vi "PixieCalcCountDataold.vi"(0 "CrsrList":T2, 1 "Histogram Data":u32[][](array[numeric]), 2 "CH0 LT":dbl, 3 "CH1 LT":dbl) -> (5 "Count Data":T1)   [LabVIEW 2011]
uses:
  <vilib>/Utility/miscctls.llb/LVCursorListTypeDef.ctl
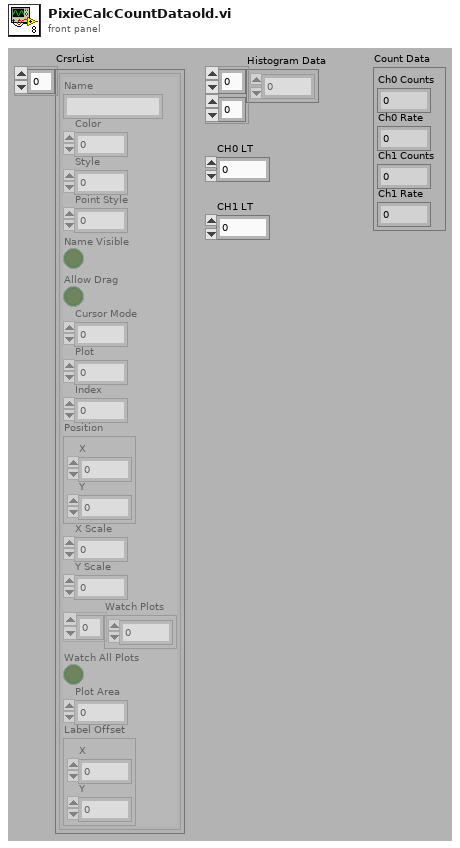
[diagram p1: front panel]
types:
  T1 = cluster{"Ch0 Counts":u32, "Ch0 Rate":dbl, "Ch1 Counts":u32, "Ch1 Rate":dbl}
  T2 = typedef "LVCursorListTypeDef.ctl" = cluster{"Name":string, "Color":u32, "Style":u8, "Point Style":u8, "Name Visible":bool, "Allow Drag":bool, "Cursor Mode":u32, "Plot":i32, "Index":i32, "Position":cluster{"X":dbl, "Y":dbl}, "X Scale":u32, "Y Scale":u32, "Watch Plots":i32[], "Watch All Plots":bool, "Plot Area":i32, "Label Offset":cluster{"X":dbl, "Y":dbl}}[]
  T3 = cluster{"Name":string, "Color":u32, "Style":u8, "Point Style":u8, "Name Visible":bool, "Allow Drag":bool, "Cursor Mode":u32, "Plot":i32, "Index":i32, "Position":cluster{"X":dbl, "Y":dbl}, "X Scale":u32, "Y Scale":u32, "Watch Plots":i32[], "Watch All Plots":bool, "Plot Area":i32, "Label Offset":cluster{"X":dbl, "Y":dbl}}
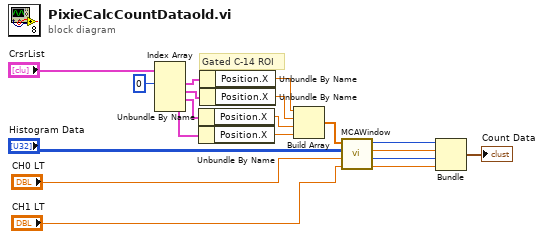
[diagram p0: block diagram]
diagram:
  # "Gated C-14 ROI"
  n1 = Index Array(array="CrsrList", index #1=0 ("index")) -> (element #1=w10:T3, element #2=w11:T3, element #3=w12:T3, element #4=w13:T3)  [unwired: 3 in]
  n2 = Unbundle By Name(w12) -> ("Position.X"=w3:dbl)
  n3 = Unbundle By Name(w13) -> ("Position.X"=w5:dbl)
  n4 = Unbundle By Name(w10) -> ("Position.X"=w7:dbl)
  n5 = Unbundle By Name(w11) -> ("Position.X"=w6:dbl)
  n6 = Build Array(w7, w6, w3, w5) -> (w4:dbl[])
  n7 = call "MCAWindow.vi"("Ch1 Livetime"="CH1 LT", "Ch0 Livetime"="CH0 LT", "Histogram Data"="Histogram Data", "Window"=w4) -> ("Ch1 Rate"=w17:dbl, "Ch1 Counts"=w16:u32, "Ch0 Rate"=w15:dbl, "Ch0 Counts"=w14:u32)  [unwired: 4 out]
  n8 = Bundle("Ch0 Counts"=w14, "Ch0 Rate"=w15, "Ch1 Counts"=w16, "Ch1 Rate"=w17) -> (→"Count Data":T1)  [unwired: 1 out]
